vi "CalculateBounds.vi"(7 "menu in":refnum<class "menu.lvclass">, 8 "error in (no error)":errorcluster, 11 "text item in":refnum<class "text item.lvclass">) -> (0 "error out":errorcluster, 2 "bounds":cluster{"width":u32, "height":u32}, 3 "text item out":refnum<class "text item.lvclass">)   [LabVIEW 2009, in "text item.lvclass"]
uses:
  text item.lvclass
  Menu/menu.lvclass
  text item.lvclass/text item.ctl
  Text/text.lvclass
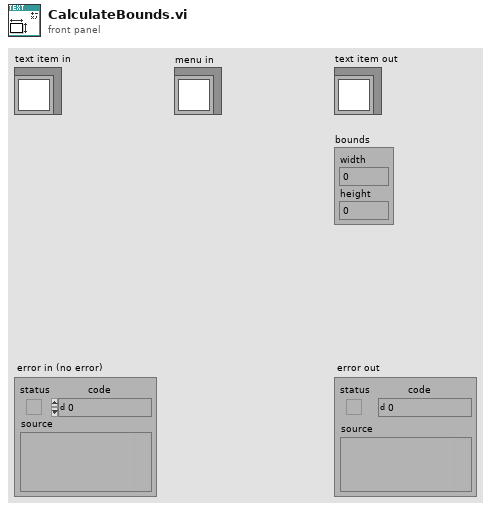
[diagram p1: front panel]
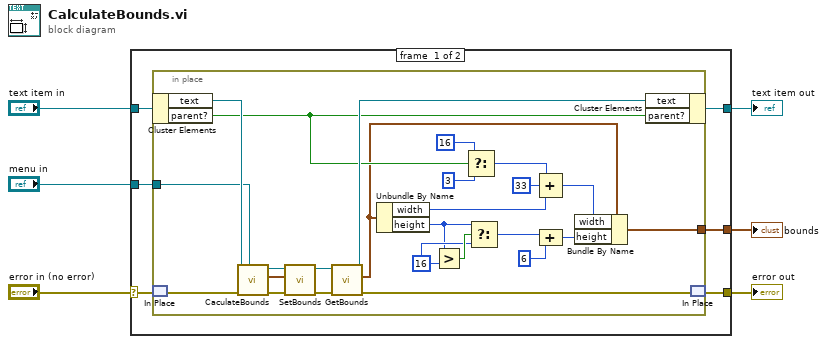
[diagram p0: block diagram]
diagram:
  n1 = case shown="No Error" "error in (no error)" {
    selector: "error in (no error)" -> [w10 w39]
    tunnel: [w9 w39] -> w3
    tunnel: [w11 w38] -> w5
    tunnel: "text item in" -> [w12 w38]
    tunnel: "menu in" -> [w8 _]
    tunnel: [w7 _] -> w1
    frame #0 {
      n2 = in-place {
        in-place-border: w8 -> [w32]
        in-place-border: [w13] -> w7
        w26 = u32 16 ("y")
        n3 = in-place-cluster #1(w12) -> ("text"=w35:refnum<class "text.lvclass">, "parent?"=w20:bool)
        n4 = in-place-match #2(w10) -> (w37:errorcluster)
        n5 = call "CaculateBounds.vi"("menu in"=w32, "error in (no error)"=w37, "text in"=w35) -> ("error out"=w34:errorcluster, "bounds"=w33:cluster{"width":u32, "height":u32}, "text out"=w36:refnum<class "text.lvclass">)  [unwired: 6 in]
        n6 = call "SetBounds.vi"("error in (no error)"=w34, "bounds"=w33, "text in"=w36) -> ("error out"=w30:errorcluster, "text out"=w31:refnum<class "text.lvclass">)  [unwired: 7 in]
        n7 = call "GetBounds.vi"("error in (no error)"=w30, "text in"=w31) -> ("error out"=w28:errorcluster, "bounds"=w14:cluster{"width":u32, "height":u32}, "text out"=w29:refnum<class "text.lvclass">)  [unwired: 7 in]
        n8 = Unbundle By Name(w14) -> ("width"=w23:u32, "height"=w25:u32)
        n9 = Greater?(x=w25, y=w26) -> (0:w27:bool)
        n10 = Select(t=u32 16 ("value"), s=w20, f=u32 3 ("value")) -> (s? t:f=w17:u32)
        n11 = Select(t=w25, s=w27, f=w26) -> (s? t:f=w24:u32)
        n12 = Compound Arithmetic op=ADD(w17, u32 33 ("value"), w23) -> (w22:u32)
        n13 = Compound Arithmetic op=ADD(w24, u32 6 ("value")) -> (w16:u32)
        n14 = Bundle By Name(cluster=w14, "width"=w22, "height"=w16) -> (w13:cluster{"width":u32, "height":u32})
        n15 = in-place-cluster #1("text"=w29, "parent?"=w20) -> (w11:refnum<class "text item.lvclass">)
        n16 = in-place-match #2(w28) -> (w9:errorcluster)
      }
    }
    frame #1 {
    }
  }
  "text item out" <- w5
  "error out" <- w3
  "bounds" <- w1
